vi "Read from Buffer.vi"   [LabVIEW 2017, in "Waveforms (N Ch).lvclass"]
doc: "Adds buffering to stimulus-response applications. You must manually select the polymorphic instance to use."
uses:
  <vilib>/addons/_NISVFA/_Shared subVIs/Data Objects/Waveforms (DBL)/Waveforms (N Ch).lvclass
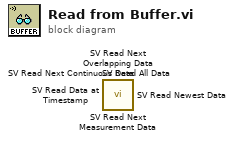
[diagram p0: block diagram]
diagram:
  n1 = call <vilib>:"SV Read Next Measurement Data.vi"() -> ()  [unwired: 7 in, 5 out]
  n2 = call <vilib>:"SV Read All Data.vi"() -> ()  [unwired: 9 in, 3 out]
  n3 = call <vilib>:"SV Read Data at Timestamp.vi"() -> ()  [unwired: 8 in, 4 out]
  n4 = call <vilib>:"SV Read Newest Data.vi"() -> ()  [unwired: 8 in, 4 out]
  n5 = call <vilib>:"SV Read Next Overlapping Data.vi"() -> ()  [unwired: 8 in, 4 out]
  n6 = call <vilib>:"SV Read Next Continuous Data.vi"() -> ()  [unwired: 8 in, 4 out]
